vi "Instantiate_llm_gemini.vi"(0 "model_name":string(combo), 5 "Gemini_api_key":string, 11 "error in (no error)":errorcluster) -> (4 "llm_openai out":refnum<class "llm_gemini_chatmodels.lvclass">, 15 "error out":errorcluster)   [LabVIEW 2020, in "llm_gemini_chatmodels.lvclass"]
uses:
  llm_gemini_chatmodels.lvclass
  D:/Personal/LabVIEW LLMs/src/models/abstract_llm_base/abstract_llm_base.lvclass
  llm_gemini_chatmodels.lvclass/llm_gemini_chatmodels.ctl
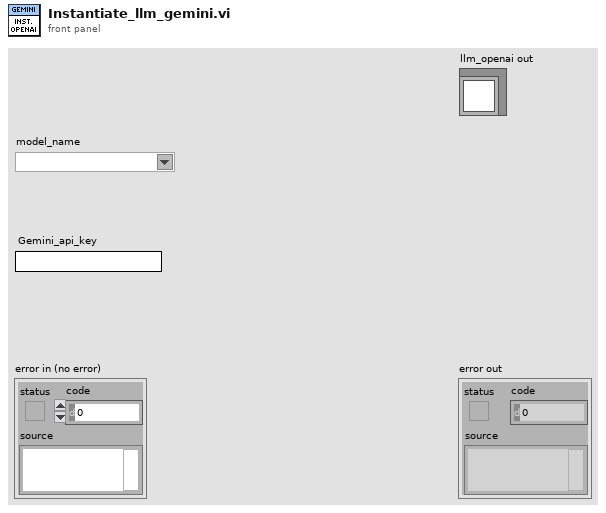
[diagram p1: front panel]
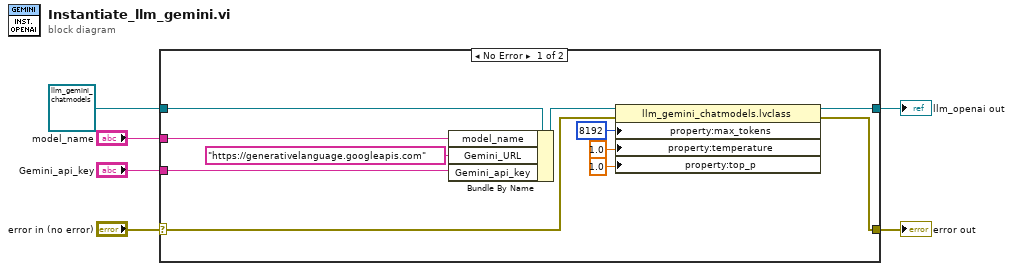
[diagram p0: block diagram]
diagram:
  n1 = case shown="No Error" "error in (no error)" {
    selector: "error in (no error)" -> [w11 w19]
    tunnel: [w10 w19] -> w5
    tunnel: [w12 w18] -> w3
    tunnel: refnum<class "llm_gemini_chatmodels.lvclass"> refnum ("llm_openai in") -> [w17 w18]
    tunnel: "model_name" -> [w16 _]
    tunnel: "Gemini_api_key" -> [w14 _]
    frame No Error {
      n2 = Bundle By Name(cluster=w17, "model_name"=w16, "Gemini_URL"="https://generativelanguage.googleapis.com" ("OpenAI_URL"), "Gemini_api_key"=w14) -> (w13:refnum<class "llm_gemini_chatmodels.lvclass">)
      n3 = property class="llm_gemini_chatmodels.lvclass"(reference=w13, error in=w11, "property:max_tokens"=u32 8192 ("max_tokens"), "property:temperature"=1.0 ("temperature"), "property:top_p"=1.0 ("top_p")) -> (reference out=w12:refnum<class "llm_gemini_chatmodels.lvclass">, error out=w10:errorcluster)
    }
    frame Error {
    }
  }
  "error out" <- w5
  "llm_openai out" <- w3
